vi "Gyro Read.vi"(11 "I2CDevRef In":T2 {"Device Address" format="%.0x"}) -> (2 "Angular Rate":dbl, 3 "Angle":dbl)   [LabVIEW 2013]
uses:
  <vilib>/Rock Robotics/WPI/I2C/WPI_I2CDevRef.ctl
  <vilib>/Rock Robotics/SystemInterfaces/Typedef/FPGA_TypedefDigitalModule.ctl
  DPS Mode.ctl
  Gyro Globals.vi
panel:
  out "DPS Mode":T1
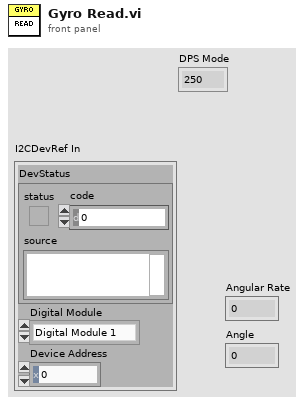
[diagram p1: front panel]
types:
  T1 = typedef "DPS Mode.ctl" = enum16{"250", "500", "2000"}
  T2 = typedef "WPI_I2CDevRef.ctl" = cluster{"DevStatus":errorcluster, "Digital Module":T3, "Device Address":u8}
  T3 = typedef "FPGA_TypedefDigitalModule.ctl" = enum16{"Digital Module 1", "Digital Module 2"}
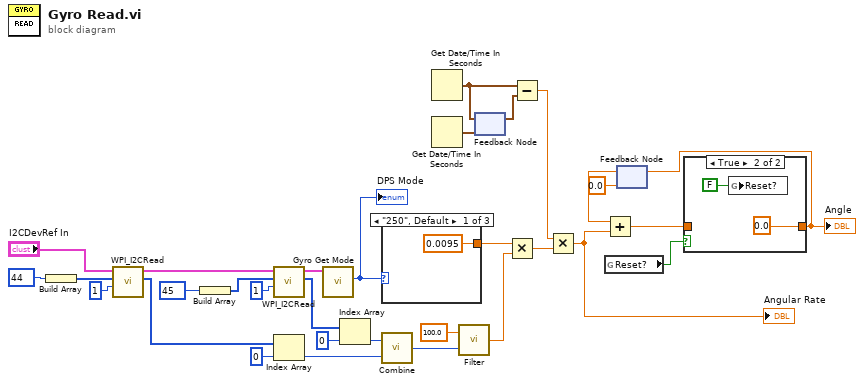
[diagram p0: block diagram]
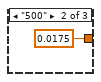
[diagram p3: hidden frame]
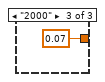
[diagram p4: hidden frame]
diagram:
  n1 = Build Array(u8 44 ("Data To Send")) -> (w31:u8[])
  n2 = call <vilib>:"WPI_I2CRead.vi"("I2CBytesToRead"=u8 1, "I2CRegister"=w31, "I2CDevRef"="I2CDevRef In") -> ("Data Out"=w24:u8[], "I2CDevRef"=w25:T2)  [unwired: 6 in, 1 out]
  n3 = Build Array(u8 45 ("Data To Send")) -> (w27:u8[])
  n4 = call <vilib>:"WPI_I2CRead.vi"("I2CBytesToRead"=u8 1, "I2CRegister"=w27, "I2CDevRef"=w25) -> ("Data Out"=w21:u8[], "I2CDevRef"=w10:T2)  [unwired: 6 in, 1 out]
  n5 = Index Array(array=w24, index=0) -> (element=w19:u8)
  n6 = call "Gyro Get Mode.vi"("I2CDevRef"=w10) -> ("DPS Mode"=w9:T1)  [unwired: 9 in, 1 out]
  "DPS Mode" <- w9
  n7 = Index Array(array=w21, index=0) -> (element=w20:u8)
  n8 = case shown="\"250\", Default" w9 {
    tunnel: [0.0095 ("Gyro Gain") 0.0175 ("Gyro Gain") 0.07 ("Gyro Gain")] -> w8
    frame "250", Default {
    }
    frame "500" {
    }
    frame "2000" {
    }
  }
  n9 = call "Combine.vi"("L"=w19, "H"=w20) -> ("Out"=w18:i16)
  n10 = Get Date/Time In Seconds() -> (seconds since 1Jan1904=w3:timestamp)
  n11 = Get Date/Time In Seconds() -> (seconds since 1Jan1904=w2:timestamp)
  n12 = call "Filter.vi"("In"=w18, "Window"=100.0) -> ("Out"=w15:dbl)
  n13 = feedback-in #1(w3) -> ()
  n14 = feedback #1(w2) -> (w4:timestamp)
  n15 = Multiply(x=w8, y=w15) -> (x*y=w16:dbl)
  n16 = Subtract(x=w3, y=w4) -> (x-y=w1:dbl)
  n17 = Multiply(x=w1, y=w16) -> (x*y=w13:dbl)
  "Angular Rate" <- w13
  n18 = global read "Gyro Globals.vi" "Reset?"() -> (w7:bool)
  n19 = feedback #2(0.0) -> (w12:dbl)
  n20 = Add(x=w12, y=w13) -> (x+y=w6:dbl)
  n21 = case shown="True" w7 {
    tunnel: w6 -> [w35 _]
    tunnel: [w35 0.0] -> w5
    frame False {
    }
    frame True {
      n22 = global write "Gyro Globals.vi" "Reset?"(FALSE ("Reset?")) -> ()
    }
  }
  "Angle" <- w5
  n23 = feedback-in #2(w5) -> ()
